vi "Gravity Loading (Trajectory).vi"(8 "error in (no error)":errorcluster, 9 "gravity":dbl[](array[numeric]), 10 "joint position trajectory":dbl[][](array[numeric]), 11 "serial arm in":refnum<class "NI_Robotics_Serial Robot Arm.lvclass">) -> (0 "error out":errorcluster, 2 "torque trajectory":dbl[][](array[numeric]), 3 "serial arm out":refnum<class "NI_Robotics_Serial Robot Arm.lvclass">)   [LabVIEW 2017, in "NI_Kinematics.lvlib"]
doc: "Calculates the torque that gravity applies to each joint of a robotic arm. Wire data to the <B>joint positions</B> input to determine the polymorphic instance to use or manually select the instance. \n\n<B>.m file:</B> gravload"
uses:
  <vilib>/robotics/Kinematics/NI_Kinematics.lvlib
  <vilib>/robotics/Kinematics/Robot/NI_Robotics_Serial Robot Arm.lvclass
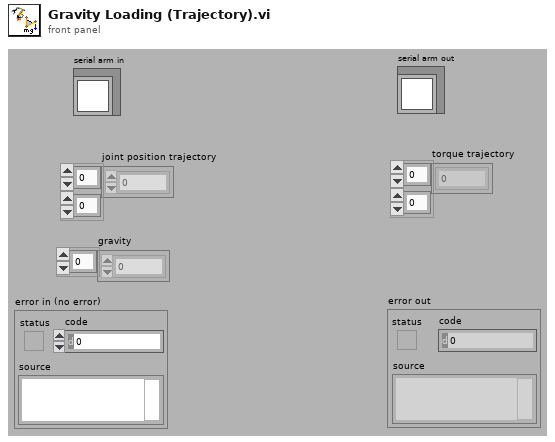
[diagram p1: front panel]
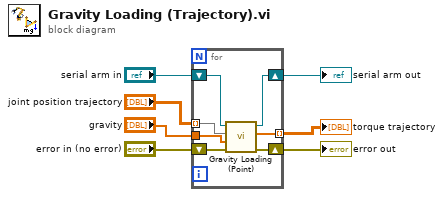
[diagram p0: block diagram]
diagram:
  n1 = for {
    tunnel: "joint position trajectory" -> [w14] mode=indexing
    tunnel: "gravity" -> [w12]
    tunnel: [w10] -> w3 mode=indexing
    shift-right: [w8] -> w1
    shift-left: "error in (no error)" -> [w9]
    shift-right: [w11] -> w4
    shift-left: "serial arm in" -> [w13]
    n2 = call <vilib>:"Gravity Loading (Point).vi"("error in (no error)"=w9, "gravity"=w12, "joint positions"=w14, "serial arm in"=w13) -> ("error out"=w8:errorcluster, "torques"=w10:dbl[], "serial arm out"=w11:refnum<class "NI_Robotics_Serial Robot Arm.lvclass">)  [unwired: 5 in]
  }
  "serial arm out" <- w4
  "torque trajectory" <- w3
  "error out" <- w1
